vi "Read Pressure and Vacuum Units.vi"(8 "error in (no error)":errorcluster, 11 "VISA resource name":refnum<visa-resource-name>) -> (0 "error out":errorcluster, 1 "Pressure Units":string, 2 "Vacuum Units":string, 3 "VISA resource name out":refnum<visa-resource-name>)   [LabVIEW 2020, in "EFD Ultimus V.lvlib"]
doc: "Reads the units the dispenser is using to display pressure and vacuum."
uses:
  EFD Ultimus V.lvlib
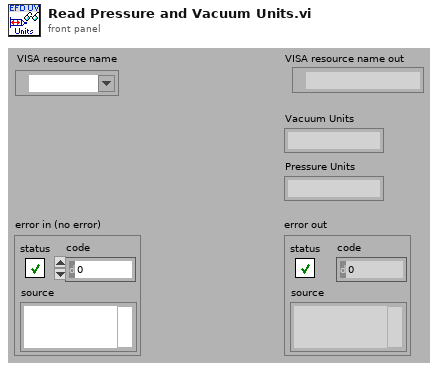
[diagram p1: front panel]
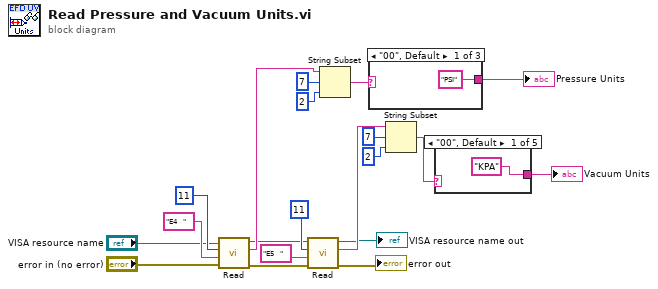
[diagram p0: block diagram]
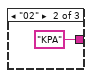
[diagram p2: hidden frame]
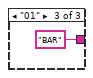
[diagram p3: hidden frame]
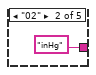
[diagram p4: hidden frame]
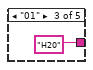
[diagram p5: hidden frame]
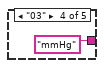
[diagram p6: hidden frame]
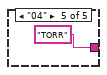
[diagram p7: hidden frame]
diagram:
  n1 = call "Read.vi"("error in (no error)"="error in (no error)", "Command To Write"="E4   ", "Bytes to Read (11)"=u32 11 ("bytes to read"), "VISA resource name"="VISA resource name") -> ("error out"=w5:errorcluster, "Ultimus V Feedback Data"=w7:string, "VISA resource name out"=w4:refnum<visa-resource-name>)  [unwired: 5 out]
  n2 = call "Read.vi"("error in (no error)"=w5, "Command To Write"="E5   ", "Bytes to Read (11)"=u32 11 ("bytes to read"), "VISA resource name"=w4) -> ("error out"=→"error out":errorcluster, "Ultimus V Feedback Data"=w18:string, "VISA resource name out"=→"VISA resource name out":refnum<visa-resource-name>)  [unwired: 5 out]
  n3 = String Subset(string=w7, offset (0)=7, length (rest)=2 ("length (rest)")) -> (substring=w8:string)
  n4 = case shown="\"00\", Default" w8 {
    tunnel: ["PSI" ("Pressure Units") "KPA" ("Pressure Units") "BAR" ("Pressure Units")] -> w3
    frame "00", Default {
    }
    frame "02" {
    }
    frame "01" {
    }
  }
  "Pressure Units" <- w3
  n5 = String Subset(string=w18, offset (0)=7, length (rest)=2 ("length (rest)")) -> (substring=w15:string)
  n6 = case shown="\"00\", Default" w15 {
    tunnel: ["KPA" ("Pressure Units") "inHg" ("Pressure Units") "H20" ("Pressure Units") "mmHg" ("Pressure Units") "TORR" ("Pressure Units")] -> w13
    frame "00", Default {
    }
    frame "02" {
    }
    frame "01" {
    }
    frame "03" {
    }
    frame "04" {
    }
  }
  "Vacuum Units" <- w13
